vi "HEWH Build States.vi"(0 "LV Program":T1, 5 "Get Gas Data":bool, 7 "Enable Ultramat 23":bool, 9 "Vesta Connect":bool) -> (4 "SM States":string)   [LabVIEW 2020]
uses:
  Utility/Save File/File Setup (Public)/Type Definition/Save File DOE LabView Program.ctl
  Utility/Save File/File Setup.lvlib
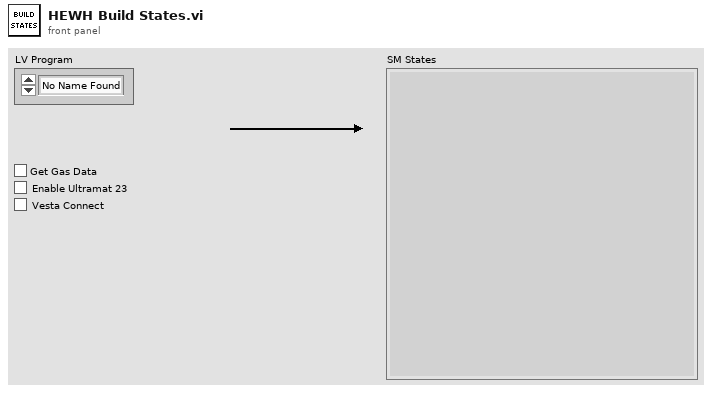
[diagram p1: front panel]
types:
  T1 = typedef "File Setup.lvlib/Save File DOE LabView Program.ctl" = enum16{"No Name Found", "DOE Stand", "Dishwasher Kitchen", "Portable Stand", "HEWH", "Dryer", "Dryer WILT", "HCC", "PRAT", "HEWH RLT", "Refrigeration", "Gas Water Heater"}
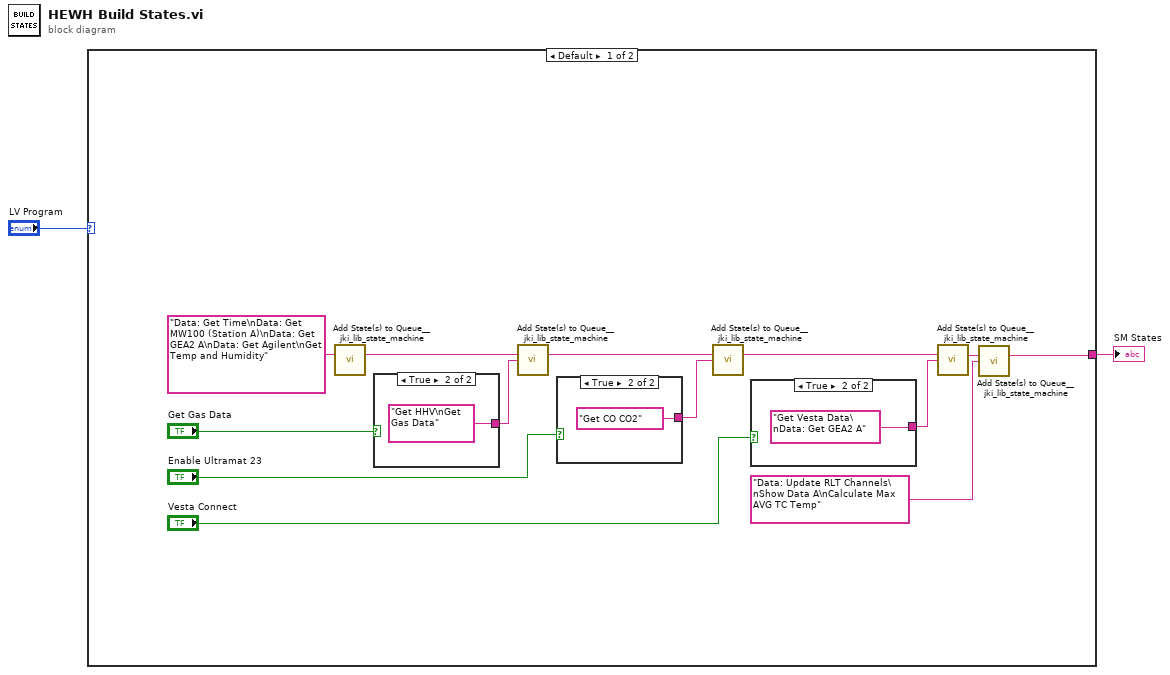
[diagram p0: block diagram]
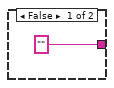
[diagram p2: hidden frame]
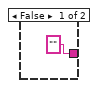
[diagram p3: hidden frame]
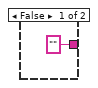
[diagram p4: hidden frame]
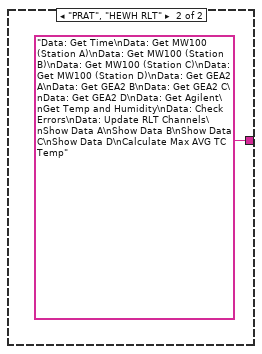
[diagram p5: hidden frame]
diagram:
  n1 = case shown="Default" "LV Program" {
    tunnel: [w3 "Data: Get Time\nData: Get MW100 (Station A)\nData: Get MW100 (Station B)\nData: Get MW100 (Station C)\nData: Get MW100 (Station D)\nData: Get GEA2 A\nData: Get GEA2 B\nData: Get GEA2 C\nData: Get GEA2 D\nData: Get Agilent\nGet Temp and Humidity\nData: Check Errors\nData: Update RLT Channels\nShow Data A\nShow Data B\nShow Data C\nShow Data D\nCalculate Max AVG TC Temp"] -> w1
    frame Default {
      n2 = call <vilib>:"Add State(s) to Queue__jki_lib_state_machine.vi"("State(s) in (\"\")"="Data: Get Time\nData: Get MW100 (Station A)\nData: Get GEA2 A\nData: Get Agilent\nGet Temp and Humidity") -> ("States Out"=w7:string)  [unwired: 14 in]
      n3 = case shown="True" "Get Gas Data" {
        tunnel: ["" "Get HHV\nGet Gas Data"] -> w9
        frame False {
        }
        frame True {
        }
      }
      n4 = call <vilib>:"Add State(s) to Queue__jki_lib_state_machine.vi"("State(s) in (\"\")"=w7, "State(s) at Back (\"\")"=w9) -> ("States Out"=w8:string)  [unwired: 13 in]
      n5 = case shown="True" "Enable Ultramat 23" {
        tunnel: ["" "Get CO CO2"] -> w6
        frame False {
        }
        frame True {
        }
      }
      n6 = call <vilib>:"Add State(s) to Queue__jki_lib_state_machine.vi"("State(s) in (\"\")"=w8, "State(s) at Back (\"\")"=w6) -> ("States Out"=w12:string)  [unwired: 13 in]
      n7 = case shown="True" "Vesta Connect" {
        tunnel: ["" "Get Vesta Data\nData: Get GEA2 A"] -> w15
        frame False {
        }
        frame True {
        }
      }
      n8 = call <vilib>:"Add State(s) to Queue__jki_lib_state_machine.vi"("State(s) in (\"\")"=w12, "State(s) at Back (\"\")"=w15) -> ("States Out"=w13:string)  [unwired: 13 in]
      n9 = call <vilib>:"Add State(s) to Queue__jki_lib_state_machine.vi"("State(s) in (\"\")"=w13, "State(s) at Back (\"\")"="Data: Update RLT Channels\nShow Data A\nCalculate Max AVG TC Temp") -> ("States Out"=w3:string)  [unwired: 13 in]
    }
    frame "PRAT", "HEWH RLT" {
    }
  }
  "SM States" <- w1
